vi "Get VS Channel References.vi"(8 "error in (no error)":errorcluster, 9 "Access (Read)":T5, 10 "Channel Refs":T1[](array[typedef]) format="%.0x", 11 "Device Reference in":T1 format="%.0x") -> (0 "error out":errorcluster, 2 "DataRef":T4 {"Block Data Refs"."Data Reference" format="%.0x"}, 3 "Device Reference out":T1=18446744073709551615 format="%.0x")   [LabVIEW 2017, in "Shared Variables CD 2.0 Engine.lvlib"]
uses:
  <vilib>/NI Veristand/Custom Device API/Custom Device Item Ref.ctl
  <vilib>/NI Veristand/Custom Device API/Data Access Type.ctl
  <vilib>/NI Veristand/Custom Device API/Block Data Reference.ctl
  <vilib>/NI Veristand/Custom Device API/Data Reference.ctl
  Shared Variables CD 2.0 Engine.lvlib
  <vilib>/NI Veristand/Custom Device API/Custom Device API.lvlib
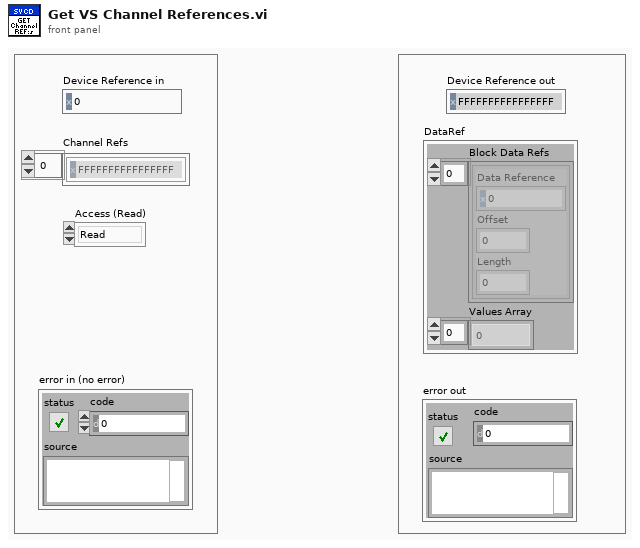
[diagram p1: front panel]
types:
  T1 = typedef "Custom Device API.lvlib/Custom Device Item Ref.ctl" = u64
  T2 = typedef "Custom Device API.lvlib/Block Data Reference.ctl" = cluster{"Data Reference":T3, "Offset":u64, "Length":u64}
  T3 = typedef "Custom Device API.lvlib/Data Reference.ctl" = i32
  T4 = cluster{"Block Data Refs":T2[], "Values Array":dbl[]}
  T5 = typedef "Custom Device API.lvlib/Data Access Type.ctl" = enum16{"Read", "Write"}
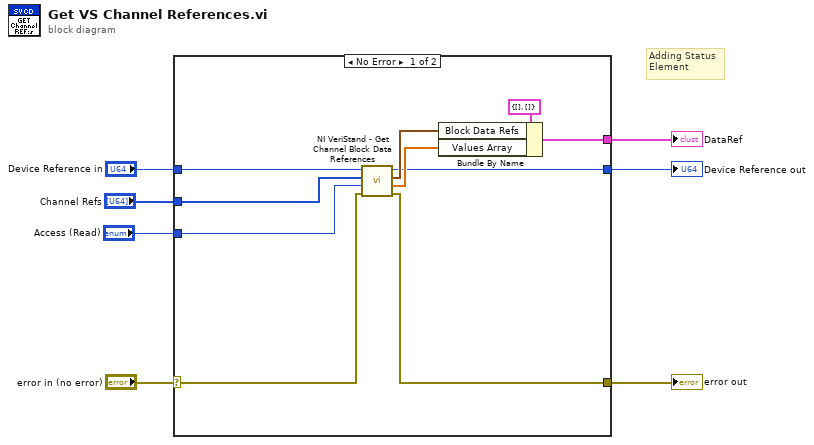
[diagram p0: block diagram]
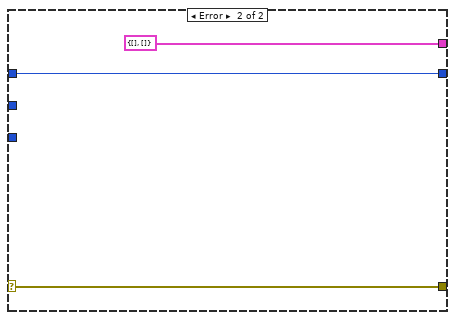
[diagram p2: hidden frame]
diagram:
  # "Adding Status\nElement"
  n1 = case shown="No Error" "error in (no error)" {
    selector: "error in (no error)" -> [w10 w20]
    tunnel: [w14 w20] -> w7
    tunnel: "Device Reference in" -> [w9 w19]
    tunnel: [w13 w19] -> w4
    tunnel: [w12 T4 {"Block Data Refs"=[], "Values Array"=[]}] -> w3
    tunnel: "Channel Refs" -> [w11 _]
    tunnel: "Access (Read)" -> [w8 _]
    frame No Error {
      n2 = call <vilib>:"NI VeriStand - Get Channel Block Data References.vi"("error in (no error)"=w10, "Access"=w8, "Channel Refs"=w11, "Device Ref in"=w9) -> ("error out"=w14:errorcluster, "Values Array"=w15:dbl[], "Block Data Refs"=w16:T2[], "Device Ref out"=w13:T1)  [unwired: 4 in]
      n3 = Bundle By Name(cluster=T4 {"Block Data Refs"=[], "Values Array"=[]}, "Block Data Refs"=w16, "Values Array"=w15) -> (w12:T4)
    }
    frame Error {
    }
  }
  "error out" <- w7
  "Device Reference out" <- w4
  "DataRef" <- w3
